vi "Enqueue Error.vi"(8 "error in":errorcluster, 11 "Error Queue":refnum<queue>) -> ()   [LabVIEW 2016]
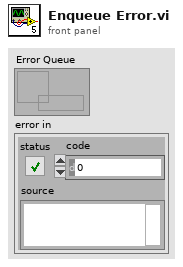
[diagram p1: front panel]
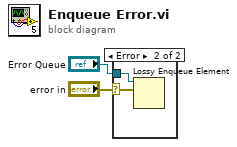
[diagram p0: block diagram]
diagram:
  n1 = case shown="Error" "error in" {
    selector: "error in" -> [_ w3]
    tunnel: "Error Queue" -> [_ w4]
    frame No Error {
    }
    frame Error {
      n2 = Lossy Enqueue Element(queue=w4, element=w3) -> ()  [unwired: 1 in, 4 out]
    }
  }
